vi "TalonSRXGetStatusRates.vi"(11 "Talon SRX DevRef In":T2={"DeviceStatus"={"status"=FALSE, "code"=0, "source"=""}, "Type"=enum."PWM", "PWM"={"PWM Channel"=enum."Invalid", "DeadBand"={"Name"="", "maxPositivePwm"=0, "minPositivePwm"=0, "centerPwm"=0, "maxNegativePwm"=0, "minNegativePwm"=0, "angularRange"=0}}, "CAN"={"Device Number"=0, "SetOutput VI Ref"=variant(enum8{"Percent VBus", "Current", "Speed", "Position", "Voltage"} enum."Percent VBus"), "GetOutput VI Ref"=variant(refnum<k1> refnum), "Enable VI Ref"=variant(dbl 12.0), "Disable VI Ref"=variant(enum8{"Percent VBus", "Speed", "Position", "Slave", "Unchanged / Invalid", "Voltage Compensation", "Current", "Motion Profile"} enum."Percent VBus"), "Data"=variant}, "Invert"=FALSE, "DIO PWM"={"PWM \"Enable\" Channel"=enum."Invalid", "DIOChannel"=enum."Invalid", "PWM Rate"=0.0}}) -> (1 "Talon SRX Get Status Rates":T1, 3 "Talon SRX DevRef Out":T2={"DeviceStatus"={"status"=FALSE, "code"=0, "source"=""}, "Type"=enum."PWM", "PWM"={"PWM Channel"=enum."Invalid", "DeadBand"={"Name"="", "maxPositivePwm"=0, "minPositivePwm"=0, "centerPwm"=0, "maxNegativePwm"=0, "minNegativePwm"=0, "angularRange"=0}}, "CAN"={"Device Number"=0, "SetOutput VI Ref"=variant(enum8{"Percent VBus", "Current", "Speed", "Position", "Voltage"} enum."Percent VBus"), "GetOutput VI Ref"=variant(refnum<k1> refnum), "Enable VI Ref"=variant(dbl 12.0), "Disable VI Ref"=variant(enum8{"Percent VBus", "Speed", "Position", "Slave", "Unchanged / Invalid", "Voltage Compensation", "Current", "Motion Profile"} enum."Percent VBus"), "Data"=variant}, "Invert"=FALSE, "DIO PWM"={"PWM \"Enable\" Channel"=enum."Invalid", "DIOChannel"=enum."Invalid", "PWM Rate"=0.0}})   [LabVIEW 2018]
uses:
  <vilib>/Rock Robotics/WPI/MotorControl/WPI_MotorControlDeviceRef.ctl
  <vilib>/Rock Robotics/WPI/MotorControl/WPI_MotorControlType.ctl
  <vilib>/Rock Robotics/SystemInterfaces/DIO/FPGA_DIOPWMChannel.ctl
  <vilib>/Rock Robotics/WPI/PWM/WPI_PWMDeadband.ctl
  <vilib>/Rock Robotics/SystemInterfaces/DIO/FPGA_DIOChannel.ctl
  <vilib>/Rock Robotics/WPI/ThirdParty/Phoenix-LabVIEW/Motor Controller/Controls/CTRE_Phoenix_MotorControl_StatusFrameEnhanced.ctl
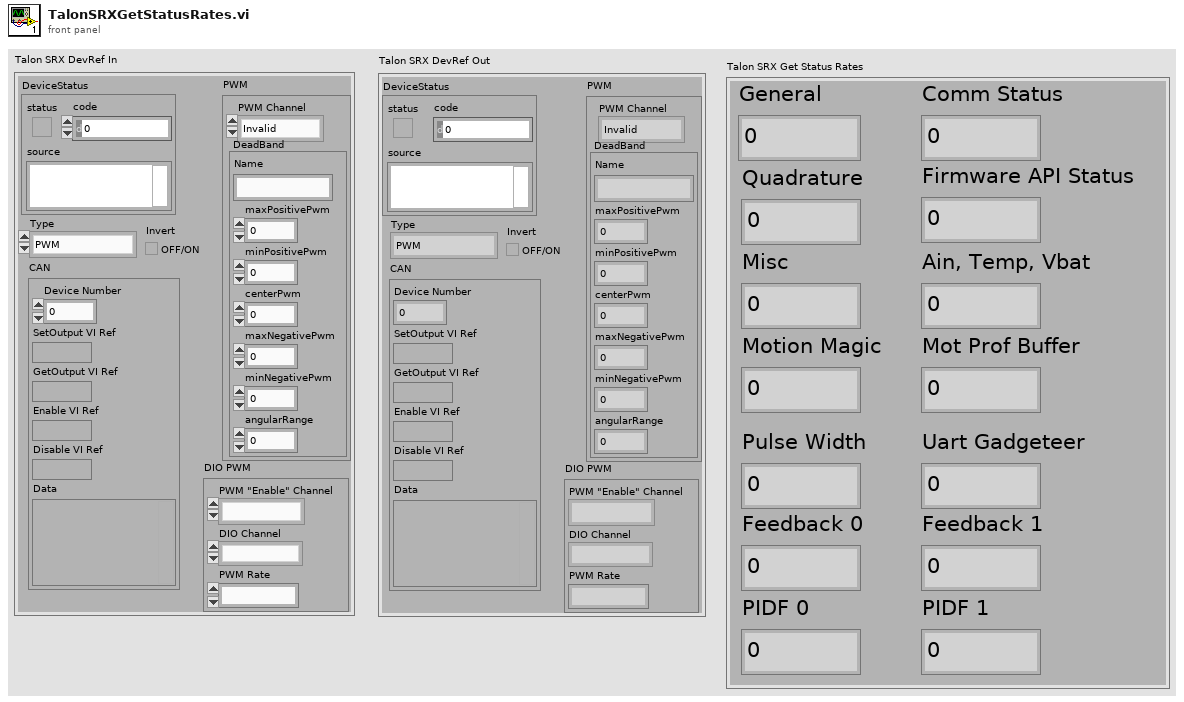
[diagram p1: front panel]
types:
  T1 = cluster{"General":u32, "Feedback 0":u32, "Quadrature":u32, "Ain, Temp, Vbat":u32, "Misc":u32, "Comm Status":u32, "PIDF 0":u32, "Feedback 1":u32, "Uart Gadgeteer":u32, "Motion Magic":u32, "Mot Prof Buffer":u32, "Pulse Width":u32, "Firmware API Status":u32, "PIDF 1":u32}
  T2 = typedef "WPI_MotorControlDeviceRef.ctl" = cluster{"DeviceStatus":errorcluster, "Type":T3, "PWM":cluster{"PWM Channel":T4, "DeadBand":T5}, "CAN":cluster{"Device Number":u8, "SetOutput VI Ref":variant, "GetOutput VI Ref":variant, "Enable VI Ref":variant, "Disable VI Ref":variant, "Data":variant}, "Invert":bool, "DIO PWM":cluster{"PWM \"Enable\" Channel":T4, "DIOChannel":T6, "PWM Rate":dbl}}
  T3 = typedef "WPI_MotorControlType.ctl" = enum16{"PWM", "CAN", "DIO PWM"}
  T4 = typedef "FPGA_DIOPWMChannel.ctl" = enum8{"PWM 0", "PWM 1", "PWM 2", "PWM 3", "PWM 4", "PWM 5", "PWM 6", "PWM 7", "PWM 8", "PWM 9", "PWM MXP 0", "PWM MXP 1", "PWM MXP 2", "PWM MXP 3", "PWM MXP 4", "PWM MXP 5", "PWM MXP 6", "PWM MXP 7", "PWM MXP 8", "PWM MXP 9", "Invalid"}
  T5 = typedef "WPI_PWMDeadband.ctl" = cluster{"Name":string, "maxPositivePwm":i32, "minPositivePwm":i32, "centerPwm":i32, "maxNegativePwm":i32, "minNegativePwm":i32, "angularRange":u16}
  T6 = typedef "FPGA_DIOChannel.ctl" = enum8{"DIO 0", "DIO 1", "DIO 2", "DIO 3", "DIO 4", "DIO 5", "DIO 6", "DIO 7", "DIO 8", "DIO 9", "DIO MXP 0", "DIO MXP 1", "DIO MXP 2", "DIO MXP 3", "DIO MXP 4", "DIO MXP 5", "DIO MXP 6", "DIO MXP 7", "DIO MXP 8", "DIO MXP 9", "DIO MXP 10", "DIO MXP 11", "DIO MXP 12", "DIO MXP 13", "DIO MXP 14", "DIO MXP 15", "SPI Port CS1", "SPI Port CS2", "SPI Port CS3", "SPI Port MISO", "SPI Port MOSI", "Invalid"}
  T7 = typedef "CTRE_Phoenix_MotorControl_StatusFrameEnhanced.ctl" = u16
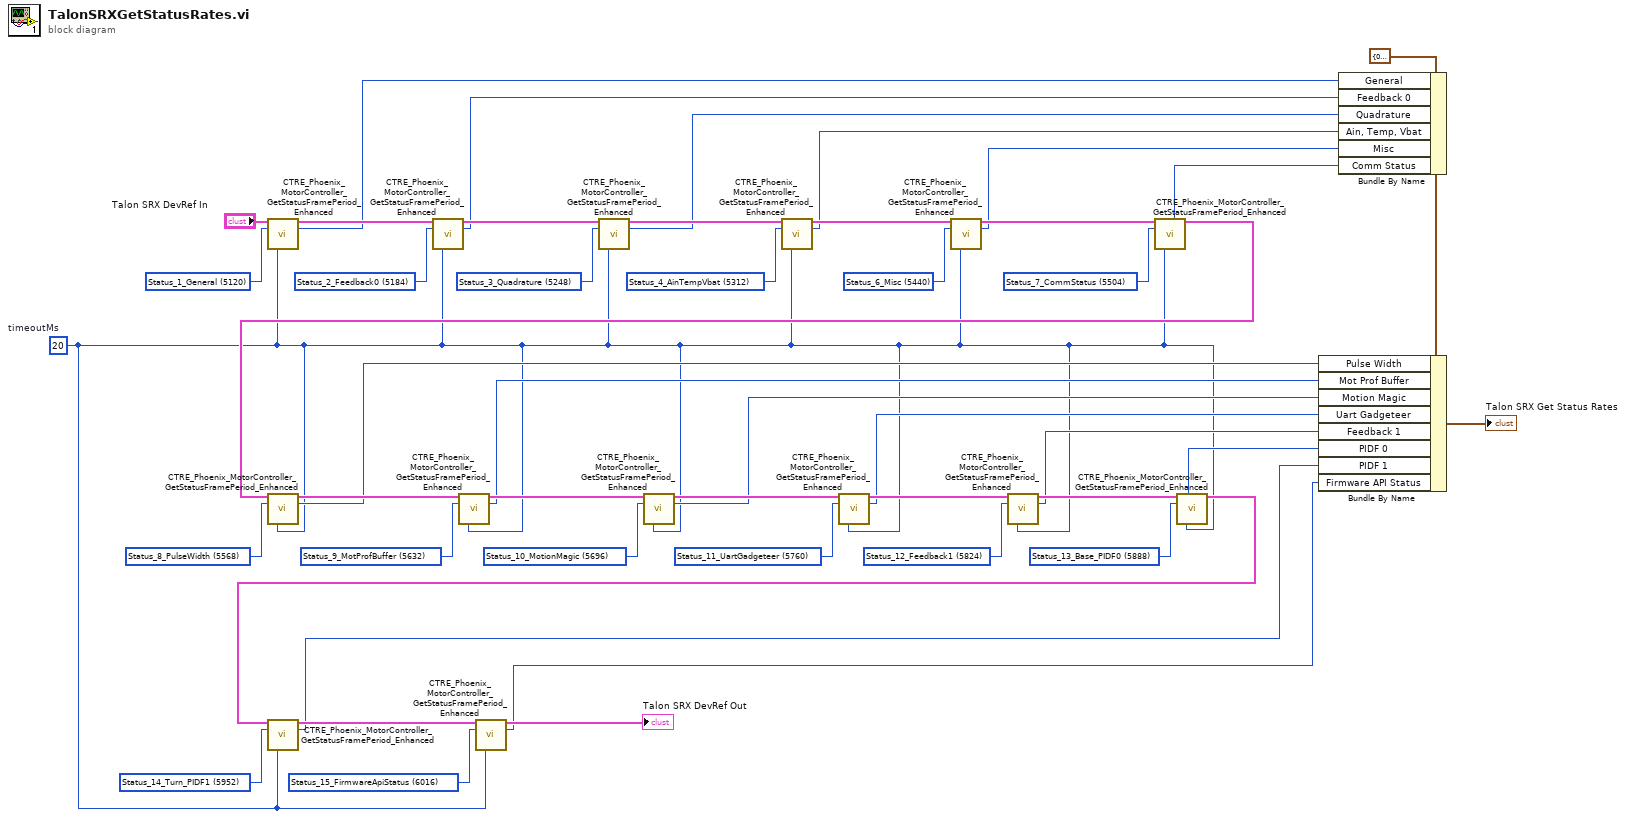
[diagram p0: block diagram]
diagram:
  w1 = u32 20  # timeoutMs
  w21 = T7 6016 items=["Status_1_General"=5120, "Status_2_Feedback0"=5184, "Status_3_Quadrature"=5248, "Status_4_AinTempVbat"=5312, "Status_6_Misc"=5440, "Status_7_CommStatus"=5504, "Status_8_PulseWidth"=5568, "Status_9_MotProfBuffer"=5632, "Status_10_MotionMagic"=5696, "Status_11_UartGadgeteer"=5760, "Status_12_Feedback1"=5824, "Status_13_Base_PIDF0"=5888, "Status_14_Turn_PIDF1"=5952, "Status_15_FirmwareApiStatus"=6016] ("Status Frame")
  w22 = T7 5952 items=["Status_1_General"=5120, "Status_2_Feedback0"=5184, "Status_3_Quadrature"=5248, "Status_4_AinTempVbat"=5312, "Status_6_Misc"=5440, "Status_7_CommStatus"=5504, "Status_8_PulseWidth"=5568, "Status_9_MotProfBuffer"=5632, "Status_10_MotionMagic"=5696, "Status_11_UartGadgeteer"=5760, "Status_12_Feedback1"=5824, "Status_13_Base_PIDF0"=5888, "Status_14_Turn_PIDF1"=5952, "Status_15_FirmwareApiStatus"=6016] ("Status Frame")
  w40 = T7 5888 items=["Status_1_General"=5120, "Status_2_Feedback0"=5184, "Status_3_Quadrature"=5248, "Status_4_AinTempVbat"=5312, "Status_6_Misc"=5440, "Status_7_CommStatus"=5504, "Status_8_PulseWidth"=5568, "Status_9_MotProfBuffer"=5632, "Status_10_MotionMagic"=5696, "Status_11_UartGadgeteer"=5760, "Status_12_Feedback1"=5824, "Status_13_Base_PIDF0"=5888, "Status_14_Turn_PIDF1"=5952, "Status_15_FirmwareApiStatus"=6016] ("Status Frame")
  w39 = T7 5824 items=["Status_1_General"=5120, "Status_2_Feedback0"=5184, "Status_3_Quadrature"=5248, "Status_4_AinTempVbat"=5312, "Status_6_Misc"=5440, "Status_7_CommStatus"=5504, "Status_8_PulseWidth"=5568, "Status_9_MotProfBuffer"=5632, "Status_10_MotionMagic"=5696, "Status_11_UartGadgeteer"=5760, "Status_12_Feedback1"=5824, "Status_13_Base_PIDF0"=5888, "Status_14_Turn_PIDF1"=5952, "Status_15_FirmwareApiStatus"=6016] ("Status Frame")
  w38 = T7 5760 items=["Status_1_General"=5120, "Status_2_Feedback0"=5184, "Status_3_Quadrature"=5248, "Status_4_AinTempVbat"=5312, "Status_6_Misc"=5440, "Status_7_CommStatus"=5504, "Status_8_PulseWidth"=5568, "Status_9_MotProfBuffer"=5632, "Status_10_MotionMagic"=5696, "Status_11_UartGadgeteer"=5760, "Status_12_Feedback1"=5824, "Status_13_Base_PIDF0"=5888, "Status_14_Turn_PIDF1"=5952, "Status_15_FirmwareApiStatus"=6016] ("Status Frame")
  w37 = T7 5696 items=["Status_1_General"=5120, "Status_2_Feedback0"=5184, "Status_3_Quadrature"=5248, "Status_4_AinTempVbat"=5312, "Status_6_Misc"=5440, "Status_7_CommStatus"=5504, "Status_8_PulseWidth"=5568, "Status_9_MotProfBuffer"=5632, "Status_10_MotionMagic"=5696, "Status_11_UartGadgeteer"=5760, "Status_12_Feedback1"=5824, "Status_13_Base_PIDF0"=5888, "Status_14_Turn_PIDF1"=5952, "Status_15_FirmwareApiStatus"=6016] ("Status Frame")
  w36 = T7 5632 items=["Status_1_General"=5120, "Status_2_Feedback0"=5184, "Status_3_Quadrature"=5248, "Status_4_AinTempVbat"=5312, "Status_6_Misc"=5440, "Status_7_CommStatus"=5504, "Status_8_PulseWidth"=5568, "Status_9_MotProfBuffer"=5632, "Status_10_MotionMagic"=5696, "Status_11_UartGadgeteer"=5760, "Status_12_Feedback1"=5824, "Status_13_Base_PIDF0"=5888, "Status_14_Turn_PIDF1"=5952, "Status_15_FirmwareApiStatus"=6016] ("Status Frame")
  w35 = T7 5568 items=["Status_1_General"=5120, "Status_2_Feedback0"=5184, "Status_3_Quadrature"=5248, "Status_4_AinTempVbat"=5312, "Status_6_Misc"=5440, "Status_7_CommStatus"=5504, "Status_8_PulseWidth"=5568, "Status_9_MotProfBuffer"=5632, "Status_10_MotionMagic"=5696, "Status_11_UartGadgeteer"=5760, "Status_12_Feedback1"=5824, "Status_13_Base_PIDF0"=5888, "Status_14_Turn_PIDF1"=5952, "Status_15_FirmwareApiStatus"=6016] ("Status Frame")
  w41 = T7 5504 items=["Status_1_General"=5120, "Status_2_Feedback0"=5184, "Status_3_Quadrature"=5248, "Status_4_AinTempVbat"=5312, "Status_6_Misc"=5440, "Status_7_CommStatus"=5504, "Status_8_PulseWidth"=5568, "Status_9_MotProfBuffer"=5632, "Status_10_MotionMagic"=5696, "Status_11_UartGadgeteer"=5760, "Status_12_Feedback1"=5824, "Status_13_Base_PIDF0"=5888, "Status_14_Turn_PIDF1"=5952, "Status_15_FirmwareApiStatus"=6016] ("Status Frame")
  w42 = T7 5440 items=["Status_1_General"=5120, "Status_2_Feedback0"=5184, "Status_3_Quadrature"=5248, "Status_4_AinTempVbat"=5312, "Status_6_Misc"=5440, "Status_7_CommStatus"=5504, "Status_8_PulseWidth"=5568, "Status_9_MotProfBuffer"=5632, "Status_10_MotionMagic"=5696, "Status_11_UartGadgeteer"=5760, "Status_12_Feedback1"=5824, "Status_13_Base_PIDF0"=5888, "Status_14_Turn_PIDF1"=5952, "Status_15_FirmwareApiStatus"=6016] ("Status Frame")
  w43 = T7 5312 items=["Status_1_General"=5120, "Status_2_Feedback0"=5184, "Status_3_Quadrature"=5248, "Status_4_AinTempVbat"=5312, "Status_6_Misc"=5440, "Status_7_CommStatus"=5504, "Status_8_PulseWidth"=5568, "Status_9_MotProfBuffer"=5632, "Status_10_MotionMagic"=5696, "Status_11_UartGadgeteer"=5760, "Status_12_Feedback1"=5824, "Status_13_Base_PIDF0"=5888, "Status_14_Turn_PIDF1"=5952, "Status_15_FirmwareApiStatus"=6016] ("Status Frame")
  w44 = T7 5248 items=["Status_1_General"=5120, "Status_2_Feedback0"=5184, "Status_3_Quadrature"=5248, "Status_4_AinTempVbat"=5312, "Status_6_Misc"=5440, "Status_7_CommStatus"=5504, "Status_8_PulseWidth"=5568, "Status_9_MotProfBuffer"=5632, "Status_10_MotionMagic"=5696, "Status_11_UartGadgeteer"=5760, "Status_12_Feedback1"=5824, "Status_13_Base_PIDF0"=5888, "Status_14_Turn_PIDF1"=5952, "Status_15_FirmwareApiStatus"=6016] ("Status Frame")
  w45 = T7 5184 items=["Status_1_General"=5120, "Status_2_Feedback0"=5184, "Status_3_Quadrature"=5248, "Status_4_AinTempVbat"=5312, "Status_6_Misc"=5440, "Status_7_CommStatus"=5504, "Status_8_PulseWidth"=5568, "Status_9_MotProfBuffer"=5632, "Status_10_MotionMagic"=5696, "Status_11_UartGadgeteer"=5760, "Status_12_Feedback1"=5824, "Status_13_Base_PIDF0"=5888, "Status_14_Turn_PIDF1"=5952, "Status_15_FirmwareApiStatus"=6016] ("Status Frame")
  w47 = T7 5120 items=["Status_1_General"=5120, "Status_2_Feedback0"=5184, "Status_3_Quadrature"=5248, "Status_4_AinTempVbat"=5312, "Status_6_Misc"=5440, "Status_7_CommStatus"=5504, "Status_8_PulseWidth"=5568, "Status_9_MotProfBuffer"=5632, "Status_10_MotionMagic"=5696, "Status_11_UartGadgeteer"=5760, "Status_12_Feedback1"=5824, "Status_13_Base_PIDF0"=5888, "Status_14_Turn_PIDF1"=5952, "Status_15_FirmwareApiStatus"=6016] ("Status Frame")
  n1 = call <vilib>:"CTRE_Phoenix_MotorController_GetStatusFramePeriod_Enhanced.vi"("PhoenixMotorControlDevRef"="Talon SRX DevRef In", "Status Frame"=w47, "timeoutMs"=w1) -> ("PhoenixMotorControlDevRef"=w29:T2, "periodMs"=w12:u32)  [unwired: 10 in, 1 out]
  n2 = call <vilib>:"CTRE_Phoenix_MotorController_GetStatusFramePeriod_Enhanced.vi"("PhoenixMotorControlDevRef"=w29, "Status Frame"=w45, "timeoutMs"=w1) -> ("PhoenixMotorControlDevRef"=w30:T2, "periodMs"=w13:u32)  [unwired: 10 in, 1 out]
  n3 = call <vilib>:"CTRE_Phoenix_MotorController_GetStatusFramePeriod_Enhanced.vi"("PhoenixMotorControlDevRef"=w30, "Status Frame"=w44, "timeoutMs"=w1) -> ("PhoenixMotorControlDevRef"=w31:T2, "periodMs"=w14:u32)  [unwired: 10 in, 1 out]
  n4 = call <vilib>:"CTRE_Phoenix_MotorController_GetStatusFramePeriod_Enhanced.vi"("PhoenixMotorControlDevRef"=w31, "Status Frame"=w43, "timeoutMs"=w1) -> ("PhoenixMotorControlDevRef"=w32:T2, "periodMs"=w15:u32)  [unwired: 10 in, 1 out]
  n5 = call <vilib>:"CTRE_Phoenix_MotorController_GetStatusFramePeriod_Enhanced.vi"("PhoenixMotorControlDevRef"=w32, "Status Frame"=w42, "timeoutMs"=w1) -> ("PhoenixMotorControlDevRef"=w33:T2, "periodMs"=w16:u32)  [unwired: 10 in, 1 out]
  n6 = call <vilib>:"CTRE_Phoenix_MotorController_GetStatusFramePeriod_Enhanced.vi"("PhoenixMotorControlDevRef"=w33, "Status Frame"=w41, "timeoutMs"=w1) -> ("PhoenixMotorControlDevRef"=w34:T2, "periodMs"=w17:u32)  [unwired: 10 in, 1 out]
  n7 = call <vilib>:"CTRE_Phoenix_MotorController_GetStatusFramePeriod_Enhanced.vi"("PhoenixMotorControlDevRef"=w34, "Status Frame"=w35, "timeoutMs"=w1) -> ("PhoenixMotorControlDevRef"=w28:T2, "periodMs"=w10:u32)  [unwired: 10 in, 1 out]
  n8 = call <vilib>:"CTRE_Phoenix_MotorController_GetStatusFramePeriod_Enhanced.vi"("PhoenixMotorControlDevRef"=w28, "Status Frame"=w36, "timeoutMs"=w1) -> ("PhoenixMotorControlDevRef"=w27:T2, "periodMs"=w9:u32)  [unwired: 10 in, 1 out]
  n9 = call <vilib>:"CTRE_Phoenix_MotorController_GetStatusFramePeriod_Enhanced.vi"("PhoenixMotorControlDevRef"=w27, "Status Frame"=w37, "timeoutMs"=w1) -> ("PhoenixMotorControlDevRef"=w26:T2, "periodMs"=w8:u32)  [unwired: 10 in, 1 out]
  n10 = call <vilib>:"CTRE_Phoenix_MotorController_GetStatusFramePeriod_Enhanced.vi"("PhoenixMotorControlDevRef"=w26, "Status Frame"=w38, "timeoutMs"=w1) -> ("PhoenixMotorControlDevRef"=w25:T2, "periodMs"=w7:u32)  [unwired: 10 in, 1 out]
  n11 = call <vilib>:"CTRE_Phoenix_MotorController_GetStatusFramePeriod_Enhanced.vi"("PhoenixMotorControlDevRef"=w25, "Status Frame"=w39, "timeoutMs"=w1) -> ("PhoenixMotorControlDevRef"=w24:T2, "periodMs"=w6:u32)  [unwired: 10 in, 1 out]
  n12 = call <vilib>:"CTRE_Phoenix_MotorController_GetStatusFramePeriod_Enhanced.vi"("PhoenixMotorControlDevRef"=w24, "Status Frame"=w40, "timeoutMs"=w1) -> ("PhoenixMotorControlDevRef"=w20:T2, "periodMs"=w5:u32)  [unwired: 10 in, 1 out]
  n13 = call <vilib>:"CTRE_Phoenix_MotorController_GetStatusFramePeriod_Enhanced.vi"("PhoenixMotorControlDevRef"=w20, "Status Frame"=w22, "timeoutMs"=w1) -> ("PhoenixMotorControlDevRef"=w23:T2, "periodMs"=w4:u32)  [unwired: 10 in, 1 out]
  n14 = call <vilib>:"CTRE_Phoenix_MotorController_GetStatusFramePeriod_Enhanced.vi"("PhoenixMotorControlDevRef"=w23, "Status Frame"=w21, "timeoutMs"=w1) -> ("PhoenixMotorControlDevRef"=→"Talon SRX DevRef Out":T2, "periodMs"=w3:u32)  [unwired: 10 in, 1 out]
  n15 = Bundle By Name(cluster=T1 {"General"=0, "Feedback 0"=0, "Quadrature"=0, "Ain, Temp, Vbat"=0, "Misc"=0, "Comm Status"=0, "PIDF 0"=0, "Feedback 1"=0, "Uart Gadgeteer"=0, "Motion Magic"=0, "Mot Prof Buffer"=0, "Pulse Width"=0, "Firmware API Status"=0, "PIDF 1"=0} ("Talon SRX Status Rates"), "General"=w12, "Feedback 0"=w13, "Quadrature"=w14, "Ain, Temp, Vbat"=w15, "Misc"=w16, "Comm Status"=w17) -> (w11:T1)
  n16 = Bundle By Name(cluster=w11, "Pulse Width"=w10, "Mot Prof Buffer"=w9, "Motion Magic"=w8, "Uart Gadgeteer"=w7, "Feedback 1"=w6, "PIDF 0"=w5, "PIDF 1"=w4, "Firmware API Status"=w3) -> (→"Talon SRX Get Status Rates":T1)
